vi "Create.vi"(5 "Line in":refnum<class "Line.lvclass">, 8 "error in (no error)":errorcluster, 10 "Hits":u32, 11 "Number":u32) -> (0 "error out":errorcluster, 3 "Line":refnum<class "Line.lvclass">)   [LabVIEW 2017, in "Cobertura.lvlib" / "Line.lvclass"]
uses:
  Line.lvclass
  Line.lvclass/Line.ctl
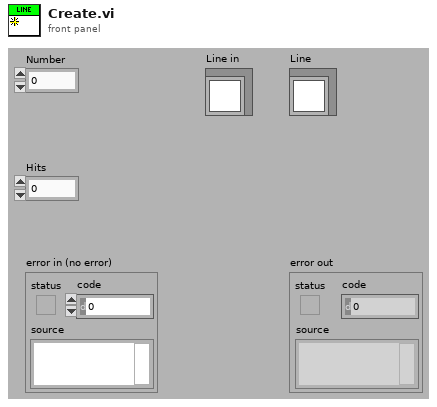
[diagram p1: front panel]
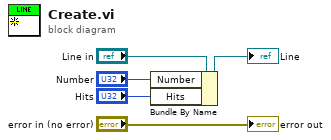
[diagram p0: block diagram]
diagram:
  n1 = Bundle By Name(cluster="Line in", "Number"="Number", "Hits"="Hits") -> (→"Line":refnum<class "Line.lvclass">)
  "error out" <- "error in (no error)"
